vi "Stop Timer.vi"(8 "error in (no error)":errorcluster, 11 "Chef Actor in":refnum<class "Chef Actor.lvclass">) -> (0 "error out":errorcluster, 3 "Chef Actor out":refnum<class "Chef Actor.lvclass">)   [LabVIEW 2024, in "Chef Actor.lvlib" / "Chef Actor.lvclass"]
uses:
  Chef Actor.lvclass
  Chef Actor.lvclass/Chef Actor.ctl
  Timer/Timer Messages/Stop Counting Msg/Stop Counting Msg.lvclass
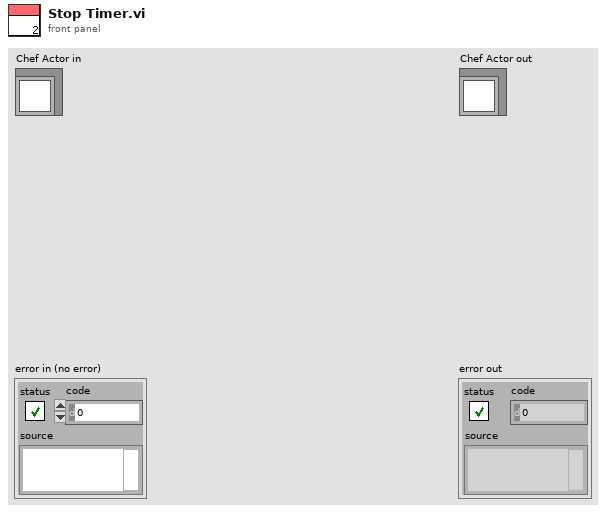
[diagram p1: front panel]
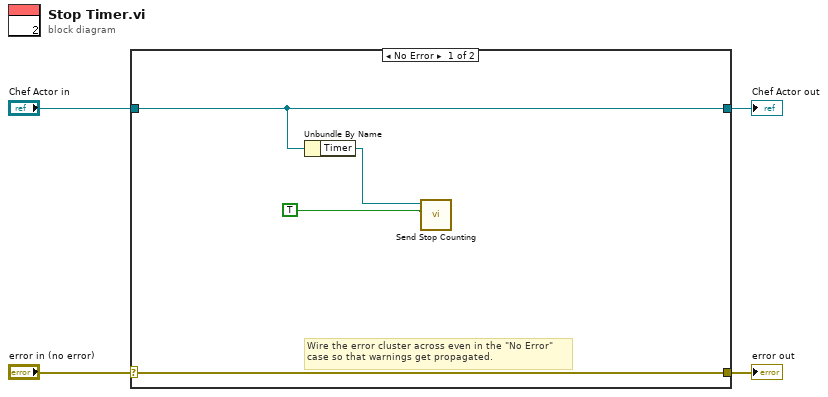
[diagram p0: block diagram]
diagram:
  n1 = case shown="No Error" "error in (no error)" {
    selector: "error in (no error)" -> [w8 w10]
    tunnel: [w8 w10] -> w3
    tunnel: [w7 w9] -> w1
    tunnel: "Chef Actor in" -> [w7 w9]
    frame No Error {
      # "Wire the error cluster across even in the \"No Error\"\ncase so that warnings get propagated."
      n2 = Unbundle By Name(w7) -> ("Timer"=w6:refnum<class "Message Enqueuer.lvclass">)
      n3 = call "Send Stop Counting.vi"("Stop?"=TRUE, "Message Enqueuer"=w6) -> ()  [unwired: 8 in, 2 out]
    }
    frame Error {
    }
  }
  "error out" <- w3
  "Chef Actor out" <- w1
